vi "参数设置页.vi"() -> ()   [LabVIEW 2016, in "斯坦道CODMn新电路板.lvlib"]
uses:
  <vilib>/Plasmionique/MB Master/MB_Master/MB_Master.lvclass
  <vilib>/ptbypt/NI_PtbyPt.lvlib
panel:
  out "error out":errorcluster
  in  "公式切换阈值滴定数(0~9999)":dbl
  in  "自动测试量程配置":T2={"水样测试量程模式"=enum."H", "标样核查量程模式"=enum."H", "零点核查量程模式"=enum."H", "跨度核查量程模式"=enum."H", "空白测试量程模式"=enum."H", "平行样测试量程模式"=enum."H", "加标回收量程模式"=enum."H", "空白校准量程模式"=enum."H", "标样校准量程模式"=enum."H"}
  out "数据刷新时间":string
  in  "通讯连接":bool
  out "MB table":enum32{"Serial", "TCP"}(tab)
  in  "请选择串口:":refnum<visa-resource-name>
  in  "IP":string="127.0.0.1"
  in  "PORT":string="1001"
  in  "通信方式选择":enum16{"串口", "TCP"}(ring)
  in  "刷新":bool
  in  "测量模式":T3(ring)
  in  "参数下拉列表":u16(ring) items=["CODMn"]
  in  "量程下拉列表":enum16{"低量程1", "低量程2", "高量程1", "高量程2"}(ring)
  in  "流程路径":path=path "data/流程.xml"
  out "阈值（高->低）":dbl caption="阈值（高->低）："
  out "阈值（低->高）":dbl caption="阈值（低->高）："
  out "量程下限":dbl caption="量程下限："
  out "量程上限":dbl caption="量程上限："
  out "检出限":dbl caption="检出限："
  out "曲线截距":dbl caption="曲线截距：" format="%#.6f"
  out "曲线斜率":dbl caption="曲线斜率：" format="%#.6f"
  out "二次多项式系数":dbl caption="二次多项式系数：" format="%#.6f"
  out "消解时长":dbl caption="消解时长："
  out "消解温度":dbl caption="消解温度："
  out "测量精度":dbl caption="测量精度："
  in  "标样核查标液浓度":dbl caption="标样核查标液浓度："
  in  "跨度核查标液浓度":dbl caption="跨度核查标液浓度："
  in  "零点核查标液浓度":dbl caption="零点核查标液浓度："
  in  "跨度值":dbl caption="跨度值："
  # "mg/L"
  # "mg/L"
  # "mg/L"
  # "mg/L"
  # "mg/L"
  # "min"
  # "℃"
  # "mg/L"
  # "mg/L"
  # "mg/L"
  # "mg/L"
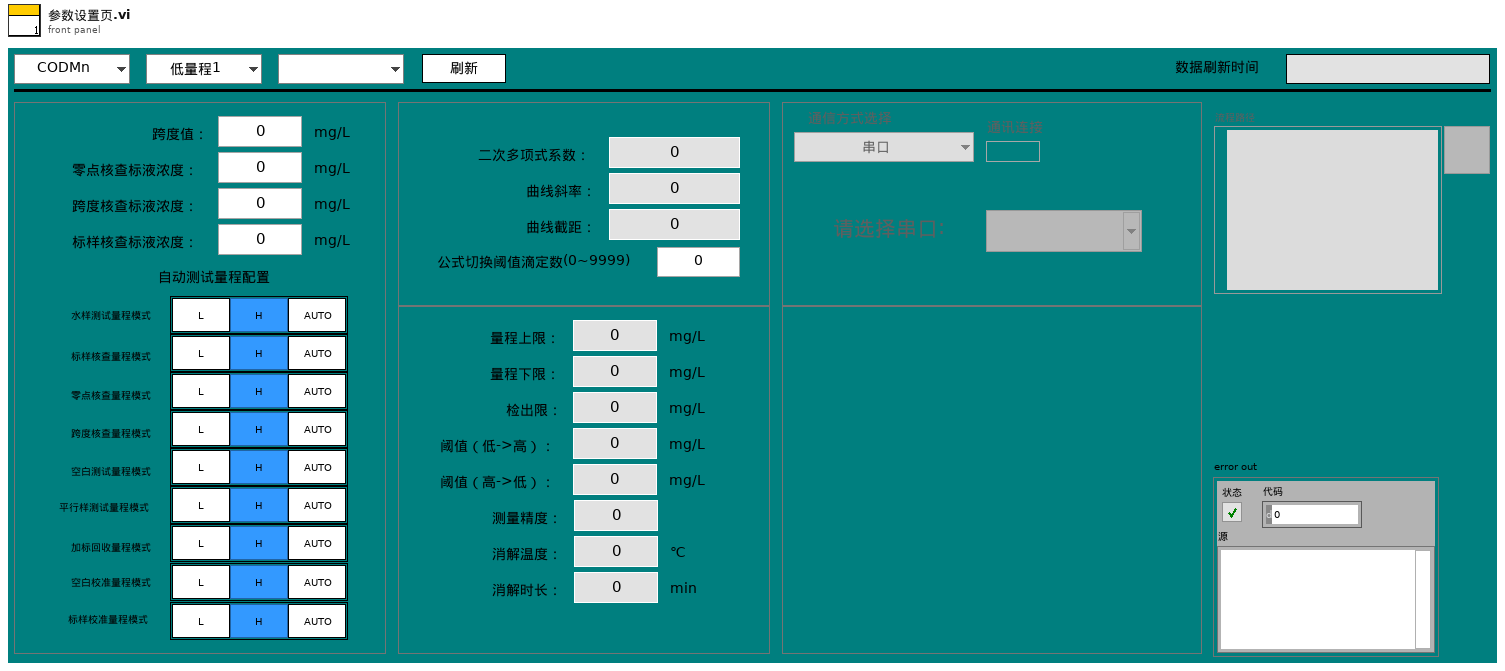
[diagram p1: front panel]
types:
  T1 = typedef "量程选择控件.ctl" = enum32{"L", "H", "AUTO"}
  T2 = cluster{"水样测试量程模式":T1, "标样核查量程模式":T1, "零点核查量程模式":T1, "跨度核查量程模式":T1, "空白测试量程模式":T1, "平行样测试量程模式":T1, "加标回收量程模式":T1, "空白校准量程模式":T1, "标样校准量程模式":T1}
  T3 = enum16{"", "水样测量", "标样核查", "零点核查", "跨度核查", "空白测试", "平行样测试", "加标回收"}
  T4 = enum8{"Enabled", "Disabled", "Disabled and Grayed Out"}
  T5 = cluster{"系统时间":timestamp, "工作状态":u16, "测量模式":enum16{"待机", "连续模式", "周期模式", "定点模式", "受控模式", "手动模式"}, "告警代码":u16, "故障代码":u16, "日志代码":u16, "软件版本":u16, "A":sgl, "B":sgl, "K":sgl, "当前滴定数":sgl, "T":sgl, "H":sgl, "id":u16, "flowid":u16, "量程":u16, "加热实时温度":sgl, "当前ORP值":sgl, "运行时间":sgl, "当前步骤剩余时间":sgl, "结束滴定数":sgl, "注射泵保温温度":sgl, "匹配滴定数X0":u16, "X^2":sgl, "X":sgl, "B 2":sgl}
  T6 = cluster{"检出限":dbl, "测量精度":dbl, "上限":dbl, "下限":dbl, "阈值（低->高）":dbl, "阈值（高->低）":dbl}
  T7 = cluster{"标液浓度1":dbl, "测量吸光度1":dbl, "样品1启用":bool, "标液浓度2":dbl, "测量吸光度2":dbl, "样品2启用":bool, "标液浓度3":dbl, "测量吸光度3":dbl, "样品3启用":bool, "标液浓度4":dbl, "测量吸光度4":dbl, "样品4启用":bool, "标液浓度5":dbl, "测量吸光度5":dbl, "样品5启用":bool, "模型":enum32{"线性", "多项式", "折线"}, "精度":dbl, "XY图":cluster{"X Values":dbl[], "Y Values":dbl[]}[], "拟合公式":string, "r^2":dbl, "标样一校准时间":timestamp, "标样二校准时间":timestamp, "标样三校准时间":timestamp, "标样四校准时间":timestamp, "标样五校准时间":timestamp, "二次方程":cluster{"c":dbl, "x":dbl, "x^2":dbl}, "标定时间":timestamp, "拟合公式 2":string, "r^2 2":dbl}[][]
  T8 = cluster{"标液浓度1":dbl, "测量吸光度1":dbl, "样品1启用":bool, "标液浓度2":dbl, "测量吸光度2":dbl, "样品2启用":bool, "标液浓度3":dbl, "测量吸光度3":dbl, "样品3启用":bool, "标液浓度4":dbl, "测量吸光度4":dbl, "样品4启用":bool, "标液浓度5":dbl, "测量吸光度5":dbl, "样品5启用":bool, "模型":enum32{"线性", "多项式", "折线"}, "精度":dbl, "XY图":cluster{"X Values":dbl[], "Y Values":dbl[]}[], "拟合公式":string, "r^2":dbl, "标样一校准时间":timestamp, "标样二校准时间":timestamp, "标样三校准时间":timestamp, "标样四校准时间":timestamp, "标样五校准时间":timestamp, "二次方程":cluster{"c":dbl, "x":dbl, "x^2":dbl}, "标定时间":timestamp, "拟合公式 2":string, "r^2 2":dbl}
  T9 = cluster{"测量量程":sgl, "测量检出限":sgl, "测量精度":sgl, "测量间隔":sgl, "消解温度":sgl, "消解时长":sgl, "三项式系数":sgl, "二次多项式系数":sgl, "曲线斜率":sgl, "曲线截距":sgl, "线性相关系数":sgl, "空白校准时间":timestamp, "标样校准时间":timestamp, "测量信号值":sgl, "稀释倍数":sgl, "量程系数":sgl}
  T10 = cluster{"偏心轮校准参数":dbl, "运行速度(修改需要重启)":u16, "加热温度(校准参数) ":dbl, "告警温度":dbl, "加热超时时间:(单位/秒)":dbl, "K p":dbl, "K i":dbl, "K d":dbl, "ILimitUp":dbl, "ILimitDown":dbl}
  T11 = cluster{"泵类型":u8, "阀数量":u8, "纯水通道":u8, "废液通道":u8, "进样速度":u16, "出样速度":u16, "滴定速度":u16, "注射泵保温温度L":u8, "注射泵保温温度H":u8, "注射泵加热超时时间":u16, "是否存在液位检测板":u16, "A值告警下限值":u16, "A值告警上限值":u16, "B值告警下限值":u16, "B值告警上限值":u16, "AB跨度告警值":u16, "阀配置:":u8}
  T12 = cluster{"跨度值":dbl, "零点标准液浓度":dbl, "跨度标准液浓度":dbl, "标准液标准浓度":dbl}
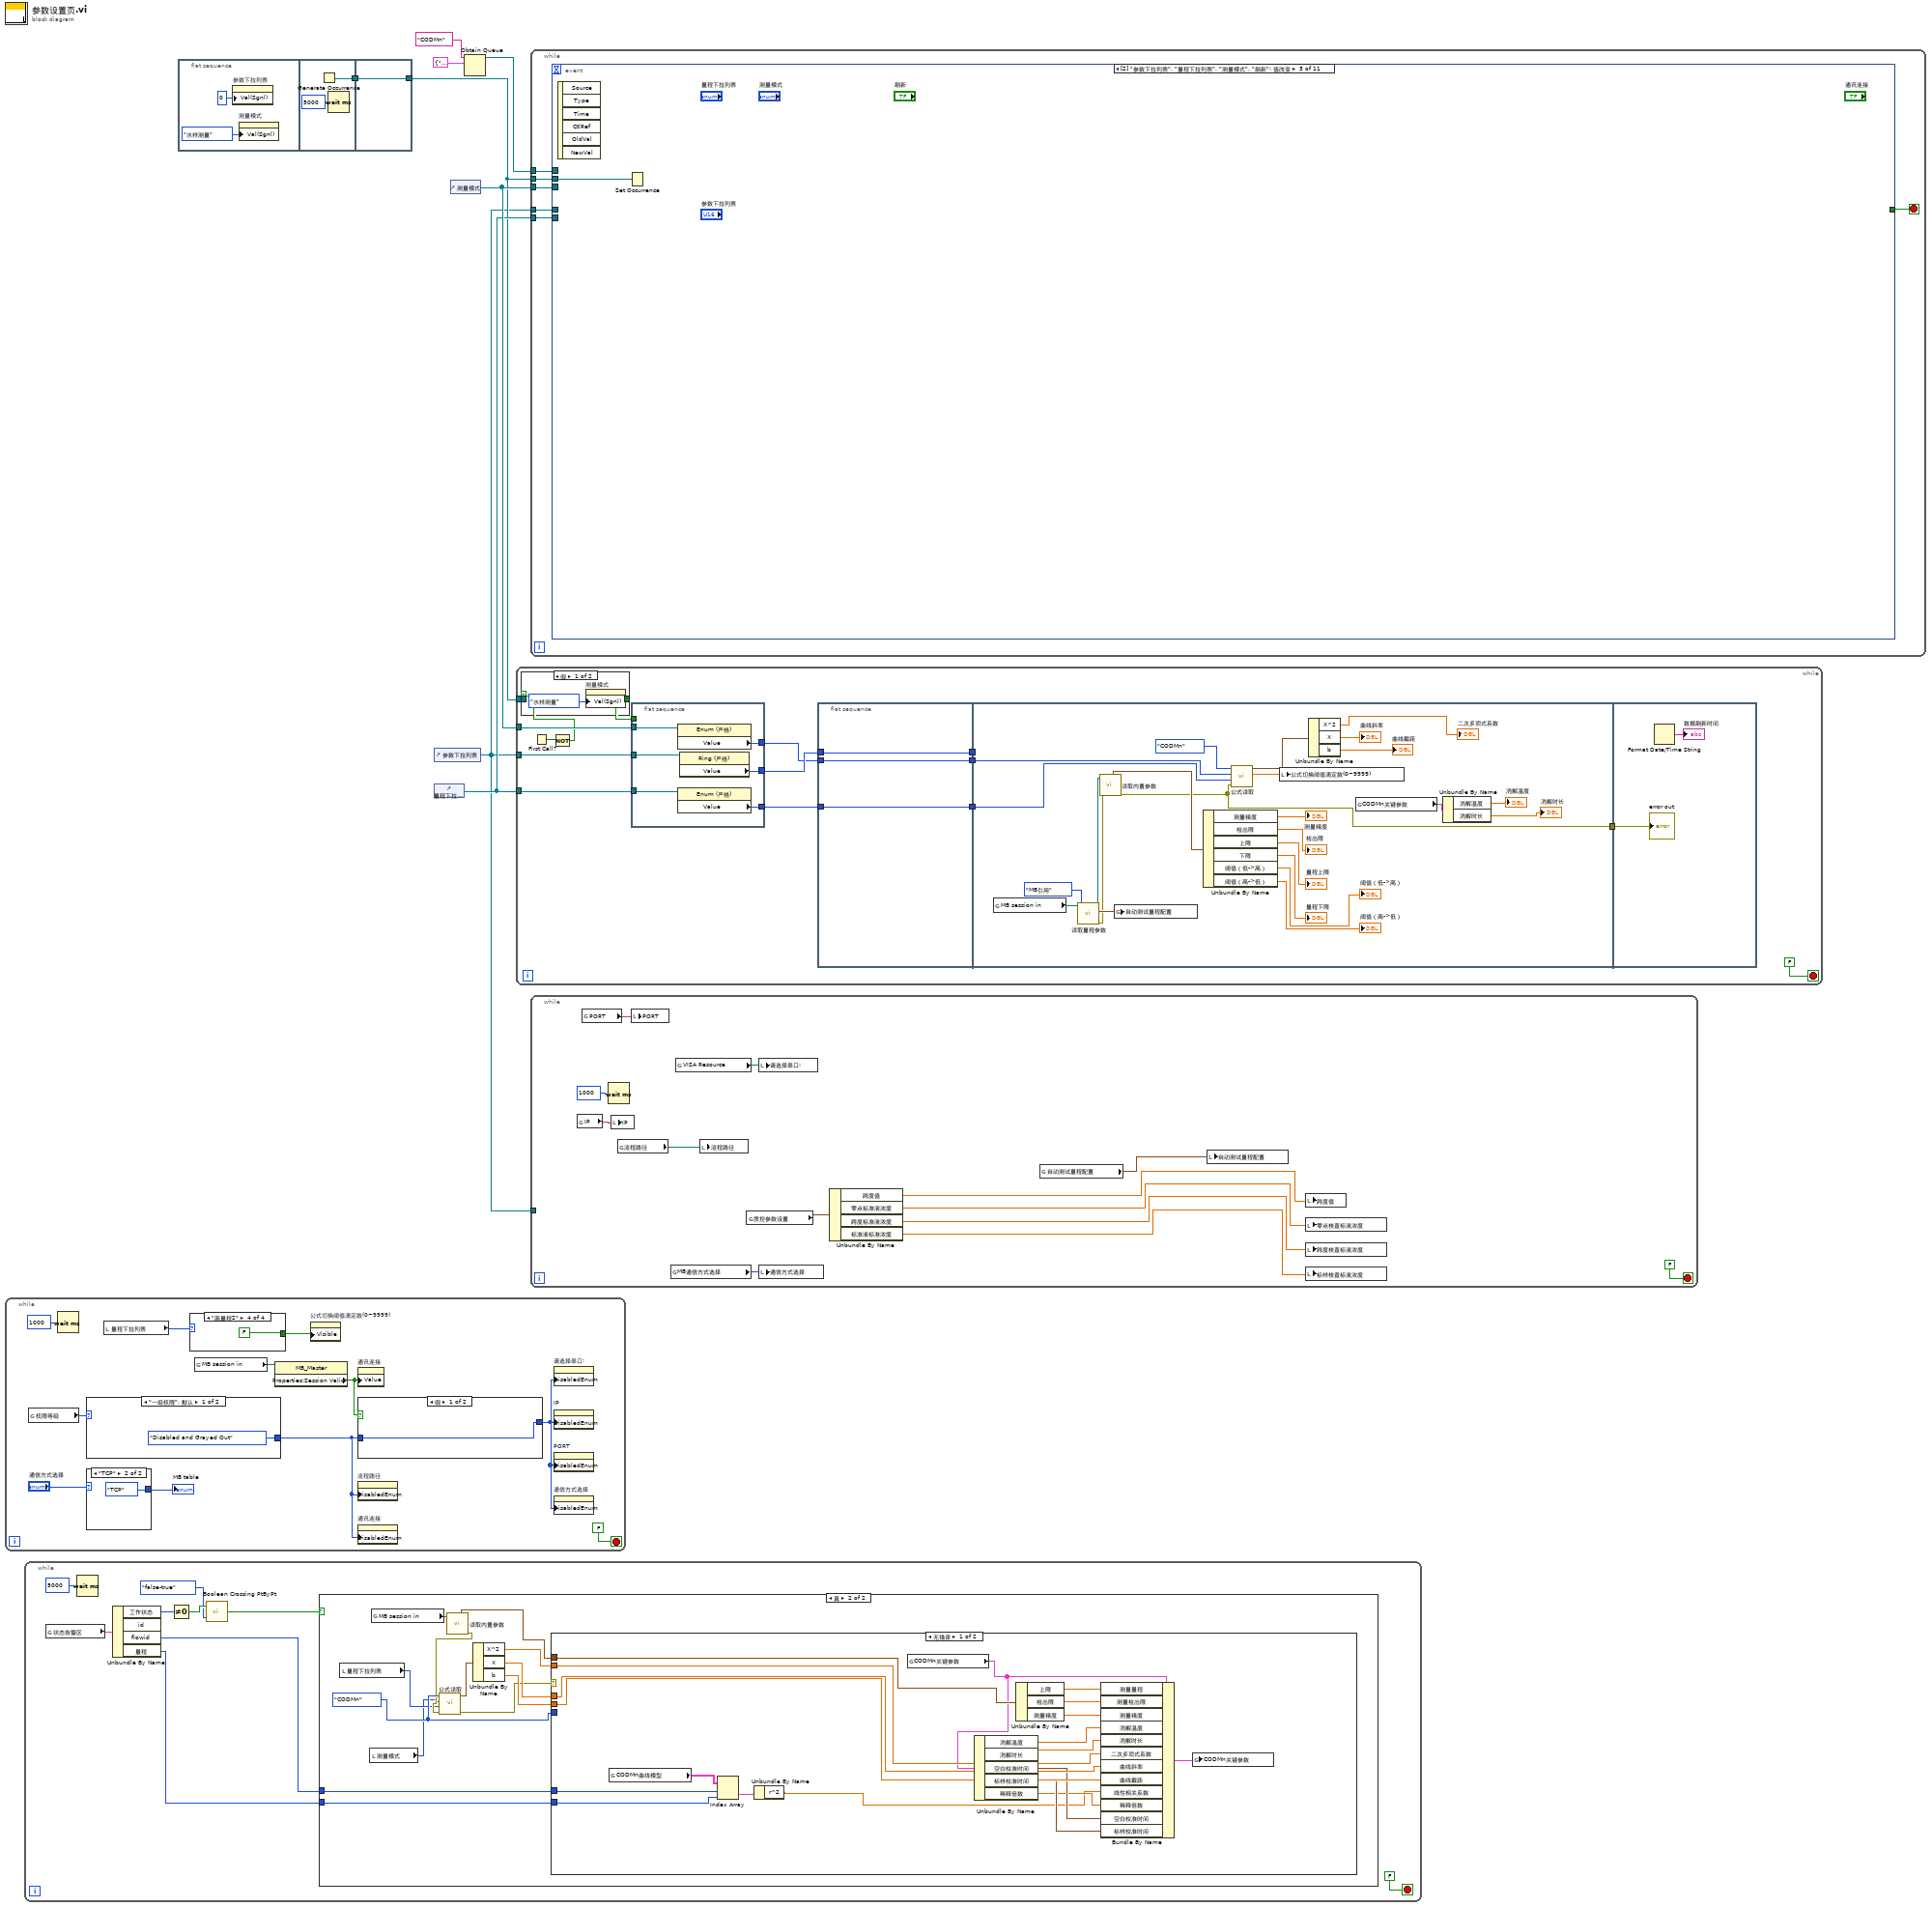
[diagram p0: block diagram]
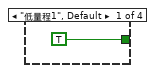
[diagram p4: hidden frame]
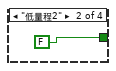
[diagram p5: hidden frame]
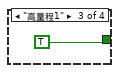
[diagram p6: hidden frame]
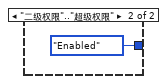
[diagram p7: hidden frame]
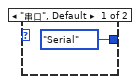
[diagram p8: hidden frame]
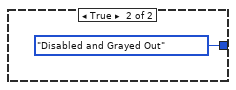
[diagram p9: hidden frame]
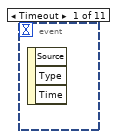
[diagram p10: hidden frame]
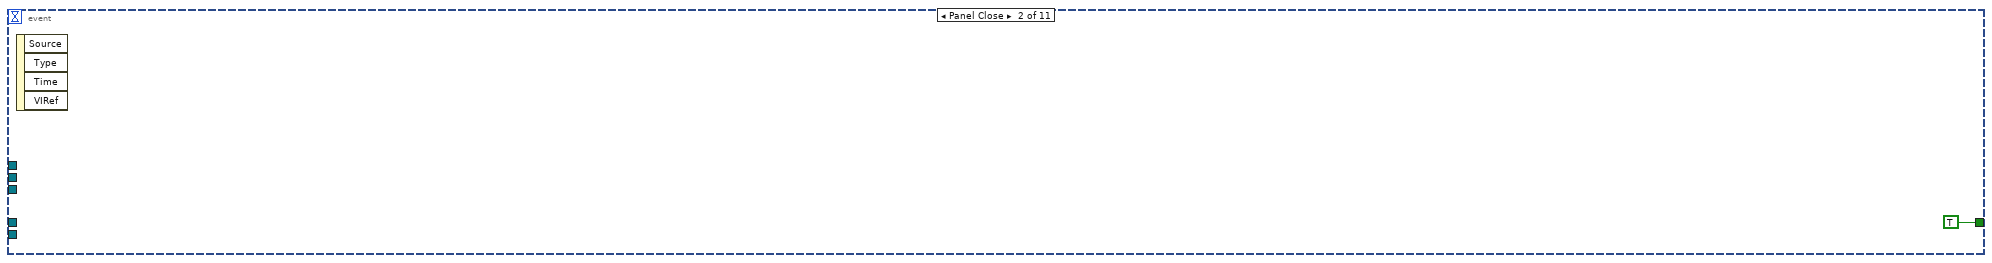
[diagram p11: hidden frame]
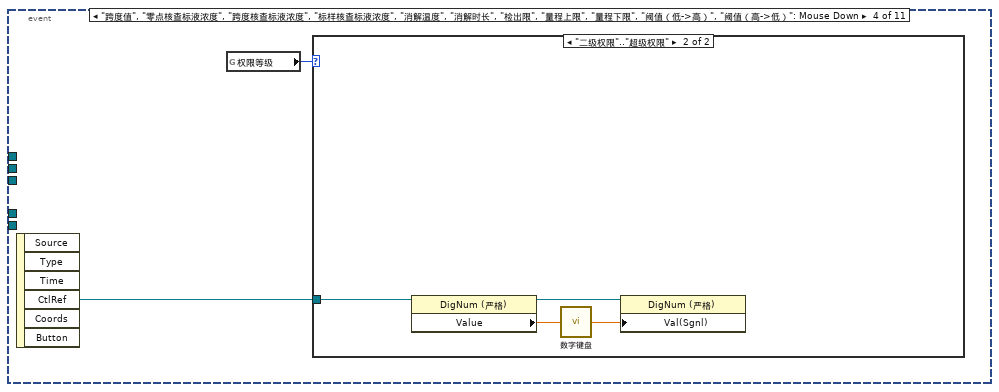
[diagram p12: hidden frame]
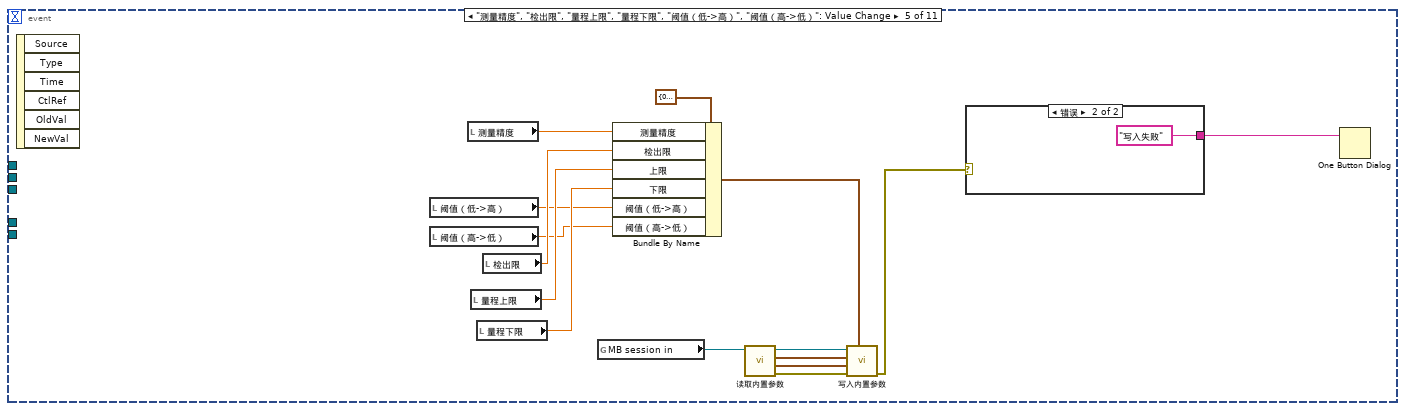
[diagram p14: hidden frame]
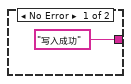
[diagram p15: hidden frame]
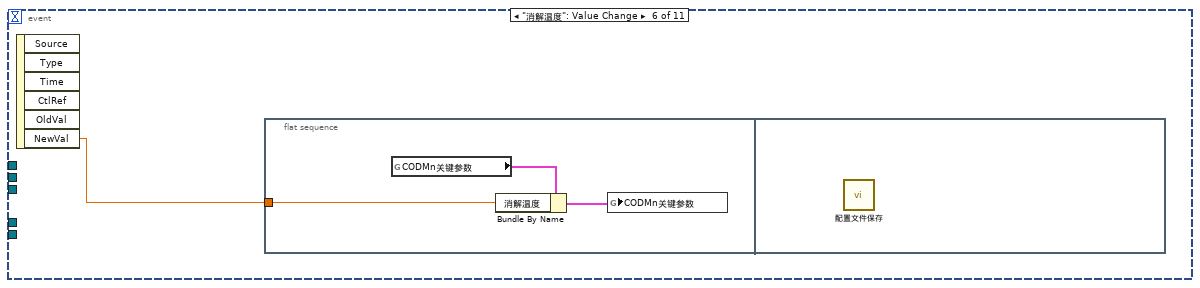
[diagram p16: hidden frame]
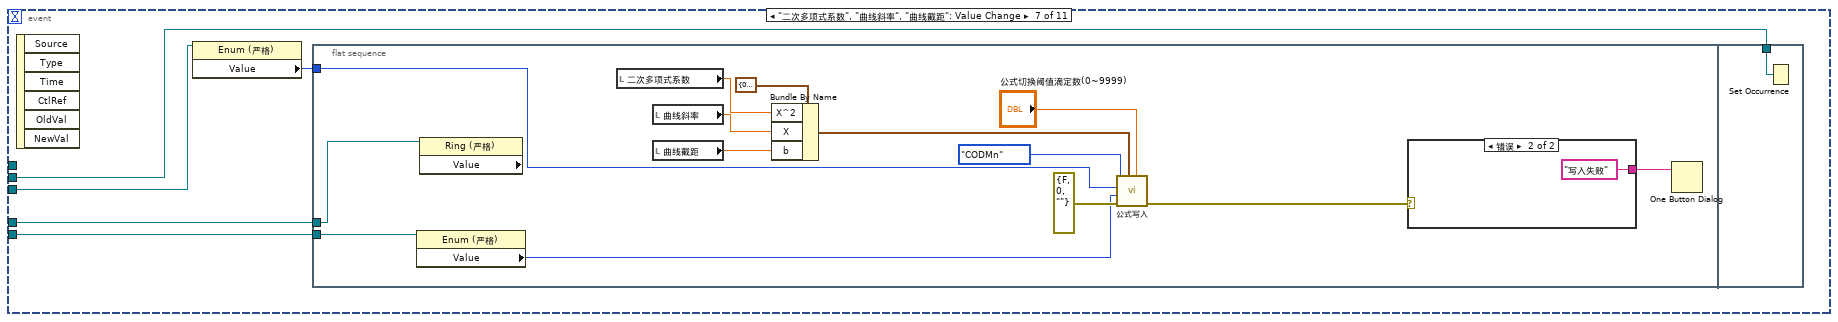
[diagram p17: hidden frame]
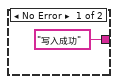
[diagram p18: hidden frame]
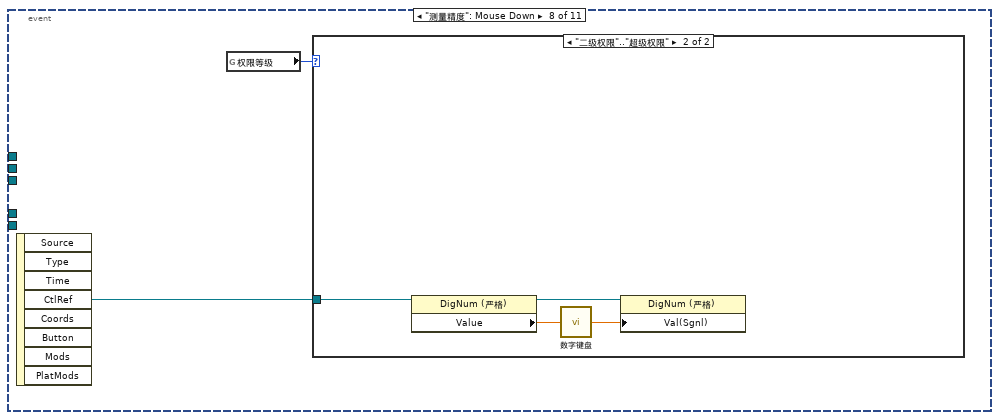
[diagram p19: hidden frame]
diagram:
  n1 = while {
    stop <- FALSE stop-if-true
    n2 = global read "VARCODMn全局变量.vi" "权限等级"() -> (w11:enum16{"一级权限", "二级权限", "三级权限", "超级权限"})
    n3 = Wait (ms)(milliseconds to wait=u32 1000 ("等待时间（毫秒）")) -> ()  [unwired: 1 out]
    n4 = case shown="\"一级权限\", 默认" w11 {
      tunnel: [T4."Disabled and Grayed Out" ("禁用") T4."Enabled" ("禁用")] -> w12
      frame "一级权限", Default {
      }
      frame "二级权限".."超级权限" {
      }
    }
    n5 = case shown="\"TCP\"" "通信方式选择" {
      tunnel: [enum32{"Serial", "TCP"}."Serial" ("MB table") enum32{"Serial", "TCP"}."TCP" ("MB table")] -> w14
      frame "串口", Default {
      }
      frame "TCP" {
      }
    }
    "MB table" <- w14
    n6 = local read "量程下拉列表"() -> (w10:enum16{"低量程1", "低量程2", "高量程1", "高量程2"})
    n7 = case shown="\"高量程2\"" w10 {
      tunnel: [TRUE FALSE TRUE FALSE] -> w9
      frame "低量程1", Default {
      }
      frame "低量程2" {
      }
      frame "高量程1" {
      }
      frame "高量程2" {
      }
    }
    n8 = global read "VARCODMn全局变量.vi" "MB session in"() -> (w18:refnum<class "MB_Master.lvclass">)
    n9 = property class="MB_Master"(reference=w18) -> ("Properties:Session Valid"=w16:bool)  [unwired: 1 in, 2 out]
    n10 = property on="公式切换阈值滴定数(0~9999)" class="DigNum (严格)"("Visible"=w9) -> ()  [unwired: 2 in, 2 out]
    n11 = property on="通讯连接" class="Bool (严格)"("Value"=w16) -> ()  [unwired: 2 in, 2 out]
    n12 = case shown="假" w16 {
      tunnel: [w28 T4."Disabled and Grayed Out" ("禁用")] -> w15
      tunnel: w12 -> [w28 _]
      frame False {
      }
      frame True {
      }
    }
    n13 = property on="流程路径" class="Path"("DisabledEnum"=w12) -> ()  [unwired: 2 in, 2 out]
    n14 = property on="通讯连接" class="Bool (严格)"("DisabledEnum"=w12) -> ()  [unwired: 2 in, 2 out]
    n15 = property on="请选择串口:" class="VISAName"("DisabledEnum"=w15) -> ()  [unwired: 2 in, 2 out]
    n16 = property on="IP" class="Str"("DisabledEnum"=w15) -> ()  [unwired: 2 in, 2 out]
    n17 = property on="PORT" class="Str"("DisabledEnum"=w15) -> ()  [unwired: 2 in, 2 out]
    n18 = property on="通信方式选择" class="Enum (严格)"("DisabledEnum"=w15) -> ()  [unwired: 2 in, 2 out]
  }
  n19 = while {
    stop <- FALSE stop-if-true
    n20 = global read "VARCODMn全局变量.vi" "状态告警区"() -> (w38:T5)
    n21 = Wait (ms)(milliseconds to wait=u32 5000 ("等待时间（毫秒）")) -> ()  [unwired: 1 out]
    n22 = Unbundle By Name(w38) -> ("工作状态"=w37:u16, "flowid"=w30:u16, "量程"=w31:u16)  [unwired: 1 out]
    n23 = Not Equal To 0?(x=w37) -> (x != 0?=w36:bool)
    n24 = call <vilib>:"Boolean Crossing PtByPt.vi"("direction"=enum16{"either", "false-true", "true-false"}."false-true", "input"=w36) -> ("crossing"=w34:bool)  [unwired: 1 in]
    n25 = case shown="真" w34 {
      tunnel: w31 -> [_ w40]
      tunnel: w30 -> [_ w39]
      frame False {
      }
      frame True {
        w47 = enum16{"CODMn"}."CODMn" ("测量参数")
        n26 = local read "量程下拉列表"() -> (w42:enum16{"低量程1", "低量程2", "高量程1", "高量程2"})
        n27 = local read "测量模式"() -> (w41:T3)
        n28 = global read "VARCODMn全局变量.vi" "MB session in"() -> (w45:refnum<class "MB_Master.lvclass">)
        n29 = call "读取内置参数.vi"("MB session in"=w45) -> ("error out"=w43:errorcluster, "量程参数读取"=w44:T6)  [unwired: 6 in, 3 out]
        n30 = call "公式读取.vi"("error in (no error)"=w43, "量程"=w42, "测量模式"=w41, "测量参数"=w47) -> ("error out"=w46:errorcluster, "公式"=w51:cluster{"X^2":dbl, "X":dbl, "b":dbl})  [unwired: 5 in, 1 out]
        n31 = Unbundle By Name(w51) -> ("X^2"=w50:dbl, "X"=w49:dbl, "b"=w48:dbl)
        n32 = case shown="无错误" w46 {
          tunnel: w44 -> [w70 _]
          tunnel: w50 -> [w69 _]
          tunnel: w49 -> [w68 _]
          tunnel: w48 -> [w67 _]
          tunnel: w47 -> [_ _]
          tunnel: w40 -> [w56 _]
          tunnel: w39 -> [w55 _]
          frame No Error {
            n33 = global read "校准数据全局变量.vi" "CODMn曲线模型"() -> (w57:T7)
            n34 = Index Array(array=w57, index (row)=w55, index (col)=w56) -> (element=w54:T8)
            n35 = Unbundle By Name(w54) -> ("r^2"=w52:dbl)
            n36 = global read "CODMn断电保存全局变量.vi" "CODMn关键参数"() -> (w59:T9)
            n37 = Unbundle By Name(w59) -> ("消解温度"=w63:sgl, "消解时长"=w62:sgl, "空白校准时间"=w60:timestamp, "标样校准时间"=w61:timestamp, "稀释倍数"=w53:sgl)
            n38 = Unbundle By Name(w70) -> ("上限"=w66:dbl, "检出限"=w65:dbl, "测量精度"=w64:dbl)
            n39 = Bundle By Name(cluster=w59, "测量量程"=w66, "测量检出限"=w65, "测量精度"=w64, "消解温度"=w63, "消解时长"=w62, "二次多项式系数"=w69, "曲线斜率"=w68, "曲线截距"=w67, "线性相关系数"=w52, "稀释倍数"=w53, "空白校准时间"=w60, "标样校准时间"=w61) -> (w58:T9)
            n40 = global write "CODMn断电保存全局变量.vi" "CODMn关键参数"(w58) -> ()
          }
          frame Error {
          }
        }
      }
    }
  }
  n41 = flat-sequence {
    tunnel: [w74] -> w8
    tunnel: [w75] -> w3
    tunnel: w8 -> [w75]
    frame #0 {
      n42 = property on="参数下拉列表" class="Ring (严格)"("Val(Sgnl)"=u16 0 ("值(信号)")) -> ()  [unwired: 2 in, 2 out]
      n43 = property on="测量模式" class="Enum (严格)"("Val(Sgnl)"=T3."水样测量" ("值(信号)")) -> ()  [unwired: 2 in, 2 out]
    }
    frame #1 {
      n44 = Generate Occurrence() -> (w74:refnum<k4>)
      n45 = Wait (ms)(milliseconds to wait=u32 5000 ("等待时间（毫秒）")) -> ()  [unwired: 1 out]
    }
    frame #2 {
    }
  }
  n46 = control-ref of="参数下拉列表"() -> (w2:refnum<vi>)
  n47 = control-ref of="量程下拉列表"() -> (w4:refnum<vi>)
  n48 = control-ref of="测量模式"() -> (w5:refnum<vi>)
  n49 = Obtain Queue(name (unnamed)="CODMn" ("名称（未命名）"), element data type=cluster{"命令":string, "data":variant} {"命令"="", "data"=variant}) -> (queue out=w6:refnum<queue>)  [unwired: 3 in, 2 out]
  n50 = while {
    tunnel: w2 -> [w89]
    tunnel: w4 -> [w88]
    tunnel: w5 -> [w87]
    tunnel: w3 -> [w86]
    stop <- FALSE stop-if-true
    n51 = First Call?() -> (First Call?: T/F=w77:bool)
    n52 = Not(x=w77) -> (.not. x?=w76:bool)
    n53 = case shown="假" w76 {
      tunnel: w86 -> [_ w93]
      tunnel: [_ w92] -> w80
      frame False {
        n54 = property on="测量模式" class="Enum (严格)"("Val(Sgnl)"=T3."水样测量" ("值(信号)")) -> ()  [unwired: 2 in, 2 out]
      }
      frame True {
        n55 = Wait on Occurrence(2:w93) -> (0:w92:bool)  [unwired: 2 in]
      }
    }
    n56 = flat-sequence {
      tunnel: w89 -> [w99]
      tunnel: w88 -> [w98]
      tunnel: w87 -> [w97]
      tunnel: [w96] -> w83
      tunnel: [w95] -> w82
      tunnel: [w94] -> w81
      tunnel: w80 -> [_]
      frame #0 {
        n57 = property class="Enum (严格)"(reference=w97) -> ("Value"=w94:T3)  [unwired: 1 in, 2 out]
        n58 = property class="Enum (严格)"(reference=w98) -> ("Value"=w95:enum16{"低量程1", "低量程2", "高量程1", "高量程2"})  [unwired: 1 in, 2 out]
        n59 = property class="Ring (严格)"(reference=w99) -> ("Value"=w96:u16)  [unwired: 1 in, 2 out]
      }
    }
    n60 = flat-sequence {
      tunnel: [w102] -> w85
      tunnel: [w101] -> w84
      tunnel: w83 -> [w100]
      tunnel: w82 -> [w102]
      tunnel: w81 -> [w101]
      tunnel: [w100] -> w78
      tunnel: w85 -> [w115]
      tunnel: w84 -> [w116]
      tunnel: [w105] -> w79
      tunnel: w78 -> [_]
      tunnel: w79 -> [w127]
      frame #0 {
      }
      frame #1 {
        n61 = global read "VARCODMn全局变量.vi" "MB session in"() -> (w109:refnum<class "MB_Master.lvclass">)
        n62 = call "读取量程参数.vi"("引用选择"=enum16{"MB引用", "自建引用"}."MB引用", "MB session in"=w109) -> ("error out"=w104:errorcluster, "自动测试量程配置"=w107:T2, "MB session out"=w103:refnum<class "MB_Master.lvclass">)  [unwired: 7 in]
        n63 = call "读取内置参数.vi"("error in (no error)"=w104, "MB session in"=w103) -> ("error out"=w105:errorcluster, "量程参数读取"=w110:T6)  [unwired: 5 in, 3 out]
        n64 = global write "CODMn断电保存全局变量.vi" "自动测试量程配置"(w107) -> ()
        n65 = Unbundle By Name(w110) -> ("测量精度"=→"测量精度":dbl, "检出限"=→"检出限":dbl, "上限"=→"量程上限":dbl, "下限"=→"量程下限":dbl, "阈值（低->高）"=→"阈值（低->高）":dbl, "阈值（高->低）"=→"阈值（高->低）":dbl)
        n66 = call "公式读取.vi"("error in (no error)"=w105, "量程"=w115, "测量模式"=w116, "测量参数"=enum16{"CODMn"}."CODMn") -> ("临界滴定数"=w112:dbl, "公式"=w120:cluster{"X^2":dbl, "X":dbl, "b":dbl})  [unwired: 5 in, 1 out]
        n67 = local write "公式切换阈值滴定数(0~9999)"(w112) -> ()
        n68 = Unbundle By Name(w120) -> ("X^2"=→"二次多项式系数":dbl, "X"=→"曲线斜率":dbl, "b"=→"曲线截距":dbl)
        n69 = global read "CODMn断电保存全局变量.vi" "CODMn关键参数"() -> (w106:T9)
        n70 = Unbundle By Name(w106) -> ("消解温度"=→"消解温度":sgl, "消解时长"=→"消解时长":sgl)
      }
      frame #2 {
        n71 = Format Date/Time String() -> (date/time string=→"数据刷新时间":string)  [unwired: 3 in]
        "error out" <- w127
      }
    }
  }
  n72 = while {
    tunnel: w3 -> [w133]
    tunnel: w2 -> [w132]
    tunnel: w6 -> [w131]
    tunnel: w5 -> [w130]
    tunnel: w4 -> [w129]
    stop <- w134 stop-if-true
    n73 = event shown="[2] \"参数下拉列表\", \"量程下拉列表\", \"测量模式\", \"刷新\": 值改变" {
      selector: _ -> [_ _ _ _ _ _ _ _ _ _ _]
      dyn-events: _ -> [_ _ _ _ _ _ _ _ _ _ _]
      timeout: _ -> [_ _ _ _ _ _ _ _ _ _ _]
      tunnel: [_ TRUE _ _ _ _ _ _ _ _ _] -> w134
      tunnel: w133 -> [_ _ w136 _ _ _ w164 _ _ w199 _]
      tunnel: w132 -> [_ _ _ _ _ _ w168 _ _ w201 _]
      tunnel: w131 -> [_ _ _ _ _ _ _ _ _ _ w221]
      tunnel: w130 -> [_ _ _ _ _ _ w167 _ _ _ _]
      tunnel: w129 -> [_ _ _ _ _ _ w165 _ _ _ _]
      event Timeout {
        n74 = event-data() -> ()  [unwired: 1 in, 3 out]
      }
      event Panel Close {
        n75 = event-data() -> ()  [unwired: 1 in, 4 out]
      }
      event "参数下拉列表", "量程下拉列表", "测量模式", "刷新": Value Change {
        n76 = event-data() -> ()  [unwired: 1 in, 6 out]
        n77 = Set Occurrence(w136) -> ()
      }
      event "跨度值", "零点核查标液浓度", "跨度核查标液浓度", "标样核查标液浓度", "消解温度", "消解时长", "检出限", "量程上限", "量程下限", "阈值（低->高）", "阈值（高->低）": Mouse Down {
        n78 = event-data() -> ("CtlRef"=w138:refnum<vi>)  [unwired: 1 in, 5 out]
        n79 = global read "VARCODMn全局变量.vi" "权限等级"() -> (w137:enum16{"一级权限", "二级权限", "三级权限", "超级权限"})
        n80 = case shown="\"二级权限\"..\"超级权限\"" w137 {
          tunnel: w138 -> [_ w142]
          frame "一级权限", Default {
          }
          frame "二级权限".."超级权限" {
            n81 = property class="DigNum (严格)"(reference=w142) -> (reference out=w140:refnum<vi>, "Value"=w141:dbl)  [unwired: 1 in, 1 out]
            n82 = call "数字键盘.vi"("OldNumber"=w141) -> ("NewNumber"=w139:dbl)
            n83 = property class="DigNum (严格)"(reference=w140, "Val(Sgnl)"=w139) -> ()  [unwired: 1 in, 2 out]
          }
        }
      }
      event "测量精度", "检出限", "量程上限", "量程下限", "阈值（低->高）", "阈值（高->低）": Value Change {
        n84 = event-data() -> ()  [unwired: 1 in, 6 out]
        n85 = local read "阈值（低->高）"() -> (w154:dbl)
        n86 = local read "阈值（高->低）"() -> (w153:dbl)
        n87 = local read "测量精度"() -> (w152:dbl)
        n88 = local read "量程上限"() -> (w157:dbl)
        n89 = local read "量程下限"() -> (w156:dbl)
        n90 = local read "检出限"() -> (w155:dbl)
        n91 = global read "VARCODMn全局变量.vi" "MB session in"() -> (w150:refnum<class "MB_Master.lvclass">)
        n92 = Bundle By Name(cluster=T6 {"检出限"=0.0, "测量精度"=0.0, "上限"=0.0, "下限"=0.0, "阈值（低->高）"=0.0, "阈值（高->低）"=0.0} ("量程参数读取"), "测量精度"=w152, "检出限"=w155, "上限"=w157, "下限"=w156, "阈值（低->高）"=w154, "阈值（高->低）"=w153) -> (w143:T6)
        n93 = call "读取内置参数.vi"("MB session in"=w150) -> ("error out"=w146:errorcluster, "float"=w147:T10, "外设配置"=w148:T11, "MB session out"=w149:refnum<class "MB_Master.lvclass">)  [unwired: 6 in, 1 out]
        n94 = call "写入内置参数.vi"("量程参数读取"=w143, "error in (no error)"=w146, "float"=w147, "外设配置"=w148, "MB session in"=w149) -> ("error out"=w145:errorcluster)  [unwired: 5 in, 1 out]
        n95 = case shown="错误" w145 {
          tunnel: ["写入成功" "写入失败"] -> w151
          frame No Error {
          }
          frame Error {
          }
        }
        n96 = One Button Dialog(message=w151) -> ()  [unwired: 1 in, 1 out]
      }
      event "消解温度": Value Change {
        n97 = event-data() -> ("NewVal"=w160:dbl)  [unwired: 1 in, 5 out]
        n98 = flat-sequence {
          tunnel: w160 -> [w163]
          frame #0 {
            n99 = global read "CODMn断电保存全局变量.vi" "CODMn关键参数"() -> (w161:T9)
            n100 = Bundle By Name(cluster=w161, "消解温度"=w163) -> (w162:T9)
            n101 = global write "CODMn断电保存全局变量.vi" "CODMn关键参数"(w162) -> ()
          }
          frame #1 {
            n102 = call "配置文件保存.vi"() -> ()  [unwired: 12 in]
          }
        }
      }
      event "二次多项式系数", "曲线斜率", "曲线截距": Value Change {
        n103 = event-data() -> ()  [unwired: 1 in, 6 out]
        n104 = property class="Enum (严格)"(reference=w167) -> ("Value"=w166:T3)  [unwired: 1 in, 2 out]
        n105 = flat-sequence {
          tunnel: w168 -> [w182]
          tunnel: w166 -> [w181]
          tunnel: w165 -> [w180]
          tunnel: w164 -> [w185]
          frame #0 {
            n106 = property class="Enum (严格)"(reference=w180) -> ("Value"=w171:enum16{"低量程1", "低量程2", "高量程1", "高量程2"})  [unwired: 1 in, 2 out]
            n107 = property class="Ring (严格)" props=["Value"](reference=w182) -> ()  [unwired: 1 in, 3 out]
            n108 = local read "二次多项式系数"() -> (w177:dbl)
            n109 = local read "曲线斜率"() -> (w176:dbl)
            n110 = local read "曲线截距"() -> (w175:dbl)
            n111 = Bundle By Name(cluster=cluster{"X^2":dbl, "X":dbl, "b":dbl} {"X^2"=0.0, "X"=0.0, "b"=0.0} ("公式"), "X^2"=w177, "X"=w176, "b"=w175) -> (w178:cluster{"X^2":dbl, "X":dbl, "b":dbl})
            n112 = call "公式写入.vi"("临界滴定数"="公式切换阈值滴定数(0~9999)", "公式"=w178, "error in (no error)"=errorcluster {"status"=FALSE, "code"=0, "source"=""} ("error out"), "量程"=w171, "测量模式"=w181, "测量参数"=enum16{"CODMn"}."CODMn") -> ("error out"=w173:errorcluster)  [unwired: 5 in]
            n113 = case shown="错误" w173 {
              tunnel: ["写入成功" "写入失败"] -> w174
              frame No Error {
              }
              frame Error {
              }
            }
            n114 = One Button Dialog(message=w174) -> ()  [unwired: 1 in, 1 out]
          }
          frame #1 {
            n115 = Set Occurrence(w185) -> ()
          }
        }
      }
      event "测量精度": Mouse Down {
        n116 = event-data() -> ("CtlRef"=w187:refnum<vi>)  [unwired: 1 in, 7 out]
        n117 = global read "VARCODMn全局变量.vi" "权限等级"() -> (w186:enum16{"一级权限", "二级权限", "三级权限", "超级权限"})
        n118 = case shown="\"二级权限\"..\"超级权限\"" w186 {
          tunnel: w187 -> [_ w191]
          frame "一级权限", Default {
          }
          frame "二级权限".."超级权限" {
            n119 = property class="DigNum (严格)"(reference=w191) -> (reference out=w189:refnum<vi>, "Value"=w190:dbl)  [unwired: 1 in, 1 out]
            n120 = call "数字键盘.vi"("OldNumber"=w190) -> ("NewNumber"=w188:dbl)
            n121 = property class="DigNum (严格)"(reference=w189, "Val(Sgnl)"=w188) -> ()  [unwired: 1 in, 2 out]
          }
        }
      }
      event "二次多项式系数", "曲线斜率", "曲线截距": Mouse Down {
        n122 = event-data() -> ("CtlRef"=w192:refnum<vi>)  [unwired: 1 in, 7 out]
        n123 = disable-structure shown="启用" {
          disable-tunnel: w192 -> [w194 _]
          frame Disabled {
            n124 = global read "VARCODMn全局变量.vi" "权限等级"() -> (w193:enum16{"一级权限", "二级权限", "三级权限", "超级权限"})
            n125 = case shown="\"三级权限\", \"超级权限\"" w193 {
              tunnel: w194 -> [_ w198]
              frame "一级权限", Default {
              }
              frame "三级权限", "超级权限" {
                n126 = property class="DigNum (严格)"(reference=w198) -> (reference out=w196:refnum<vi>, "Value"=w197:dbl)  [unwired: 1 in, 1 out]
                n127 = call "数字键盘.vi"("OldNumber"=w197) -> ("NewNumber"=w195:dbl)
                n128 = property class="DigNum (严格)"(reference=w196, "Val(Sgnl)"=w195) -> ()  [unwired: 1 in, 2 out]
              }
            }
          }
          frame Enabled {
          }
        }
      }
      event "跨度值", "零点核查标液浓度", "跨度核查标液浓度", "标样核查标液浓度", "消解时长", "流程路径", "IP", "PORT", "请选择串口:", "通信方式选择", "自动测试量程配置": Value Change {
        n129 = event-data() -> ()  [unwired: 1 in, 6 out]
        n130 = global read "VARCODMn全局变量.vi" "权限等级"() -> (w200:enum16{"一级权限", "二级权限", "三级权限", "超级权限"})
        n131 = case shown="\"二级权限\"..\"超级权限\"" w200 {
          tunnel: w201 -> [_ w203]
          tunnel: w199 -> [w202 _]
          frame "一级权限", Default {
            n132 = Set Occurrence(w202) -> ()
          }
          frame "二级权限".."超级权限" {
            n133 = flat-sequence {
              tunnel: w203 -> [_]
              frame #0 {
                n134 = global write "CODMn断电保存全局变量.vi" "PORT"("PORT") -> ()
                n135 = global write "CODMn断电保存全局变量.vi" "IP"("IP") -> ()
                n136 = global write "CODMn断电保存全局变量.vi" "流程路径"("流程路径") -> ()
                n137 = local read "通信方式选择"() -> (w210:enum16{"串口", "TCP"})
                n138 = global write "CODMn断电保存全局变量.vi" "VISA Resource"("请选择串口:") -> ()
                n139 = global read "CODMn断电保存全局变量.vi" "质控参数设置"() -> (w214:T12)
                n140 = global write "CODMn断电保存全局变量.vi" "MB通信方式选择"(w210) -> ()
                n141 = local read "消解时长"() -> (w209:dbl)
                n142 = global read "VARCODMn全局变量.vi" "MB session in"() -> (w207:refnum<class "MB_Master.lvclass">)
                n143 = global read "CODMn断电保存全局变量.vi" "CODMn关键参数"() -> (w205:T9)
                n144 = call "写入量程参数.vi"("自动测试量程配置"="自动测试量程配置", "MB session in"=w207) -> ()  [unwired: 8 in, 2 out]
                n145 = Bundle By Name(cluster=w205, "消解时长"=w209) -> (w204:T9)
                n146 = Bundle By Name(cluster=w214, "跨度值"="跨度值", "零点标准液浓度"="零点核查标液浓度", "跨度标准液浓度"="跨度核查标液浓度", "标准液标准浓度"="标样核查标液浓度") -> (w208:T12)
                n147 = global write "CODMn断电保存全局变量.vi" "CODMn关键参数"(w204) -> ()
                n148 = global write "CODMn断电保存全局变量.vi" "自动测试量程配置"("自动测试量程配置") -> ()
                n149 = global write "CODMn断电保存全局变量.vi" "质控参数设置"(w208) -> ()
              }
              frame #1 {
                n150 = call "配置文件保存.vi"() -> ()  [unwired: 12 in]
              }
            }
          }
        }
      }
      event "通讯连接": Value Change {
        n151 = event-data() -> ("NewVal"=w220:bool)  [unwired: 1 in, 5 out]
        n152 = Flush Queue(queue=w221) -> (queue out=w222:refnum<queue>)  [unwired: 1 in, 2 out]
        n153 = case shown="真" w220 {
          tunnel: w222 -> [w223 w225]
          frame False {
            n154 = Enqueue Element(queue=w223, element=cluster{"命令":string, "data":variant} {"命令"="停用模块", "data"=variant} ("元素")) -> ()  [unwired: 2 in, 3 out]
          }
          frame True {
            n155 = Enqueue Element(queue=w225, element=cluster{"命令":string, "data":variant} {"命令"="启用模块", "data"=variant} ("元素")) -> ()  [unwired: 2 in, 3 out]
          }
        }
      }
    }
  }
  n156 = while {
    tunnel: w2 -> [_]
    stop <- FALSE stop-if-true
    n157 = global read "CODMn断电保存全局变量.vi" "IP"() -> (w235:string)
    n158 = global read "CODMn断电保存全局变量.vi" "PORT"() -> (w236:string)
    n159 = Wait (ms)(milliseconds to wait=u32 1000 ("等待时间（毫秒）")) -> ()  [unwired: 1 out]
    n160 = local write "IP"(w235) -> ()
    n161 = global read "CODMn断电保存全局变量.vi" "流程路径"() -> (w234:path)
    n162 = local write "PORT"(w236) -> ()
    n163 = global read "CODMn断电保存全局变量.vi" "MB通信方式选择"() -> (w233:enum16{"串口", "TCP"})
    n164 = global read "CODMn断电保存全局变量.vi" "VISA Resource"() -> (w237:refnum<visa-resource-name>)
    n165 = local write "流程路径"(w234) -> ()
    n166 = global read "CODMn断电保存全局变量.vi" "质控参数设置"() -> (w228:T12)
    n167 = local write "请选择串口:"(w237) -> ()
    n168 = local write "通信方式选择"(w233) -> ()
    n169 = Unbundle By Name(w228) -> ("跨度值"=w229:dbl, "零点标准液浓度"=w230:dbl, "跨度标准液浓度"=w231:dbl, "标准液标准浓度"=w232:dbl)
    n170 = global read "CODMn断电保存全局变量.vi" "自动测试量程配置"() -> (w227:T2)
    n171 = local write "自动测试量程配置"(w227) -> ()
    n172 = local write "跨度值"(w229) -> ()
    n173 = local write "零点核查标液浓度"(w230) -> ()
    n174 = local write "跨度核查标液浓度"(w231) -> ()
    n175 = local write "标样核查标液浓度"(w232) -> ()
  }
